vi "APLUS Open Reset Coil.vi"(6 "Reset WattHours":bool, 8 "error in (no error)":errorcluster, 11 "Modbus Master in":refnum<class "Modbus Master.lvclass">) -> (0 "error out":errorcluster, 3 "Modbus Master out":refnum<class "Modbus Master.lvclass">)   [LabVIEW 2019]
uses:
  <vilib>/NI/Modbus Library/API/Master/Modbus Master.lvclass
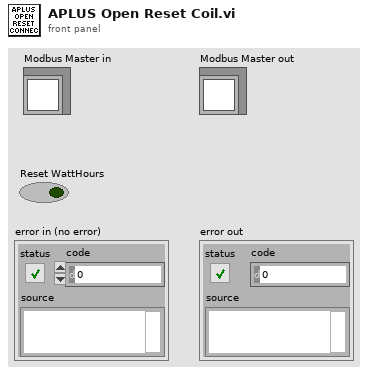
[diagram p1: front panel]
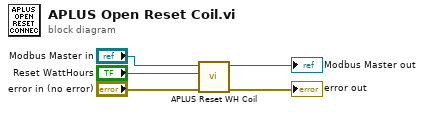
[diagram p0: block diagram]
diagram:
  n1 = call "APLUS Reset WH Coil.vi"("Error In"="error in (no error)", "Reset WattHours"="Reset WattHours", "Modbus Master in"="Modbus Master in") -> ("Error Out"=→"error out":errorcluster, "Modbus Master out"=→"Modbus Master out":refnum<class "Modbus Master.lvclass">)  [unwired: 7 in]
